vi "PLC.Dial800._TEST Set then Read Bool Value.vi"() -> ()   [LabVIEW 2018]
panel:
  in  "Write?":bool
  in  "data 2":i32
  out "data":i32
  out "Variant":variant
  out "timed out 2":bool
  out "timed out":bool
  in  "Boolean":bool
  out "timestamp":timestamp
  in  "wait for updated value (T)":bool
  in  "ms timeout (1000)":i32=1000
  out "quality":u64 format="%b"
  out "status":u32
  out "Value":bool
  out "error out":errorcluster
  in  "URL":string="opc://localhost/RSLinx OPC Server/[Stn800]Program:Stn001_90_OffloadMain.TestPC[0].Done"
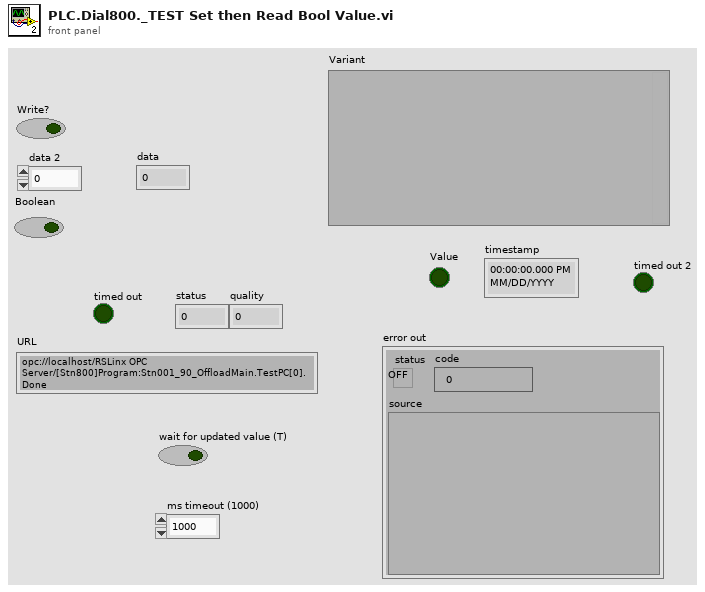
[diagram p1: front panel]
types:
  T1 = enum16{"Read", "Write", "ReadWrite", "BufferedRead", "BufferedReadWrite"}
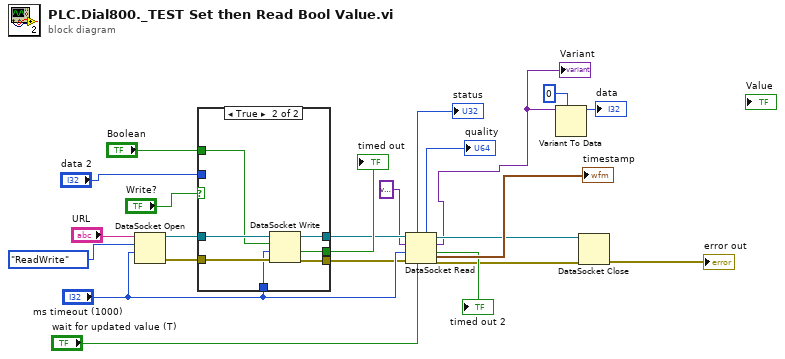
[diagram p0: block diagram]
diagram:
  n1 = DataSocket Open(9:"ms timeout (1000)", 10:T1."ReadWrite" ("mode"), 11:"URL") -> (0:w13:errorcluster, 3:w14:refnum<k13>)  [unwired: 1 in]
  n2 = case shown="True" "Write?" {
    tunnel: "Boolean" -> [_ w26]
    tunnel: [_ w32] -> w18
    tunnel: [w25 w31] -> w16
    tunnel: w14 -> [w25 w30]
    tunnel: w13 -> [w24 w29]
    tunnel: "ms timeout (1000)" -> [_ w28]
    tunnel: [w24 w27] -> w7
    tunnel: "data 2" -> [_ _]
    frame False {
    }
    frame True {
      n3 = DataSocket Write(8:w29, 9:w28, 10:w26, 11:w30) -> (0:w27:errorcluster, 1:w32:bool, 3:w31:refnum<k13>)
    }
  }
  "timed out" <- w18
  n4 = DataSocket Read(6:"wait for updated value (T)", 8:w7, 9:"ms timeout (1000)", 10:variant, 11:w16) -> (0:w11:errorcluster, 1:→"timed out 2":bool, 2:w4:variant, 3:w12:refnum<k13>, 4:→"timestamp":timestamp, 5:→"quality":u64, 7:→"status":u32)
  "Variant" <- w4
  n5 = Variant To Data(type=0, Variant=w4) -> (data=→"data":i32)  [unwired: 1 in, 1 out]
  n6 = DataSocket Close(8:w11, 11:w12) -> (0:→"error out":errorcluster)  [unwired: 1 in, 1 out]
